vi "ExecuteCommand2.vi"(11 "Command":string) -> ()   [LabVIEW 2011]
panel:
  # "The purpose of having 2 is because we sometimes need to execute a VI recursively.... this is complicated, like inception"
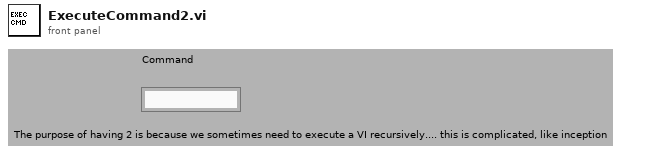
[diagram p1: front panel]
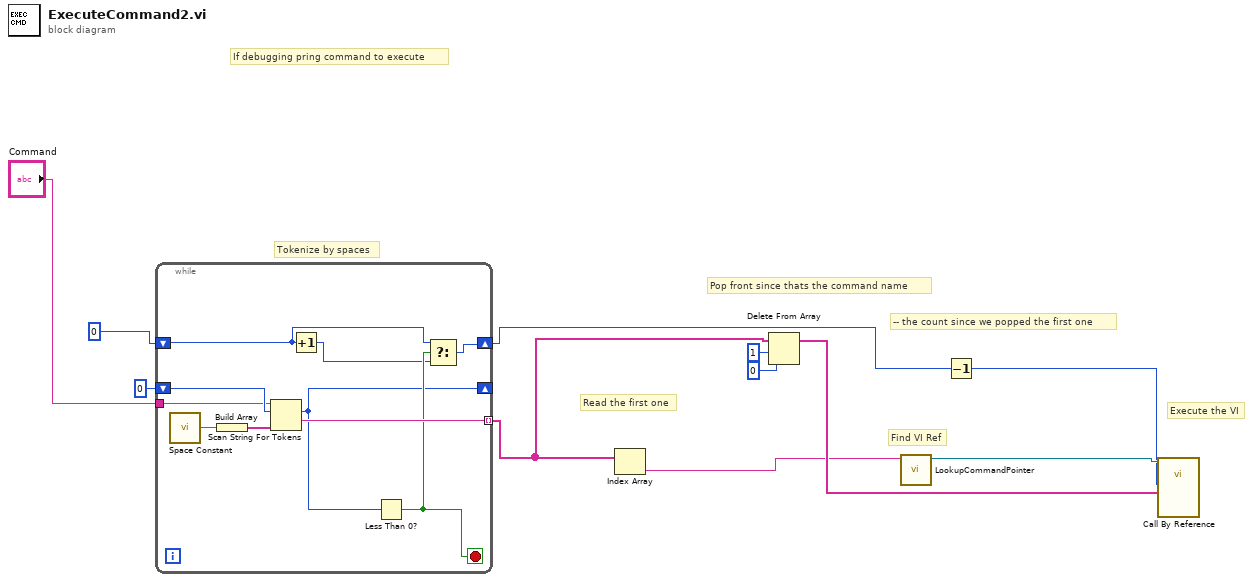
[diagram p0: block diagram]
diagram:
  # "If debugging pring command to execute"
  # "Execute the VI"
  # "-- the count since we popped the first one"
  # "Pop front since thats the command name"
  # "Find VI Ref"
  # "Read the first one"
  # "Tokenize by spaces"
  n1 = while {
    shift-right: [w12] -> _
    shift-left: 0 ("offset past token") -> [w21]
    tunnel: "Command" -> [w20]
    tunnel: [w19] -> w4 mode=indexing
    shift-right: [w15] -> w8
    shift-left: u8 0 -> [w17]
    stop <- w18 stop-if-true
    n2 = call <vilib>:"Space Constant.vi"() -> ("String"=w14:string)
    n3 = Build Array(w14) -> (w13:string[])
    n4 = Scan String For Tokens(6:w13, 8:w21, 9:w20) -> (1:w19:string, 2:w12:i32)  [unwired: 5 out]
    n5 = Increment(x=w17) -> (x+1=w16:u8)
    n6 = Less Than 0?(x=w12) -> (x < 0?=w18:bool)
    n7 = Select(t=w17, s=w18, f=w16) -> (s? t:f=w15:u8)
  }
  n8 = Index Array(array=w4) -> (element=w1:string)  [unwired: 1 in]
  n9 = Delete From Array(array=w4, length=1, index=0) -> (array with subset deleted=w5:string[])  [unwired: 1 out]
  n10 = call "LookupCommandPointer.vi"("refnum name"=w1) -> ("VI Refnum Out"=w7:refnum<vi>)  [unwired: 10 out]
  n11 = Decrement(x=w8) -> (x-1=w6:u8)
  n12 = call-by-ref "?"(reference=w7, "argv"=w5, "args"=w6) -> ()  [unwired: 11 in, 2 out]
